vi "Code_generator.vi"(1 "Code":T1(ring)) -> (0 "Array":u16[](array[numeric]) format="%b")   [LabVIEW 2018]
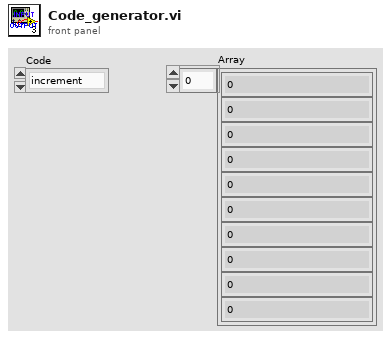
[diagram p1: front panel]
types:
  T1 = enum16{"increment", "decrement", "random", "Chess", "NChess", "One", "Zero"}
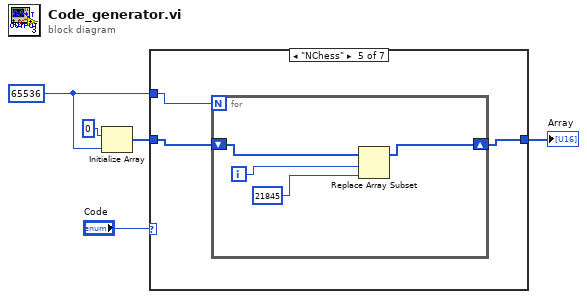
[diagram p0: block diagram]
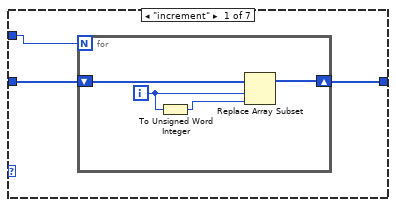
[diagram p2: hidden frame]
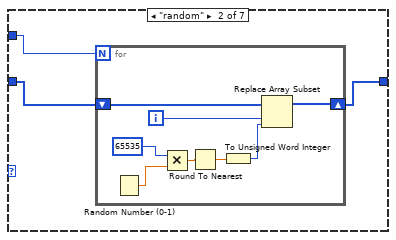
[diagram p3: hidden frame]
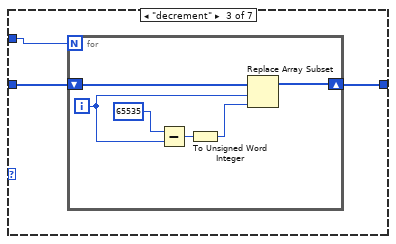
[diagram p4: hidden frame]
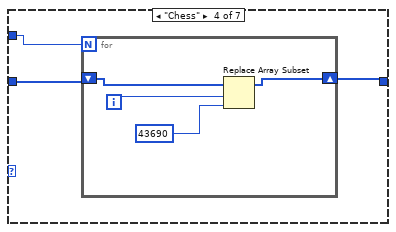
[diagram p5: hidden frame]
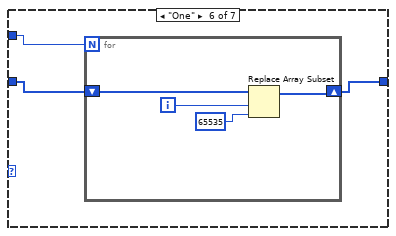
[diagram p6: hidden frame]
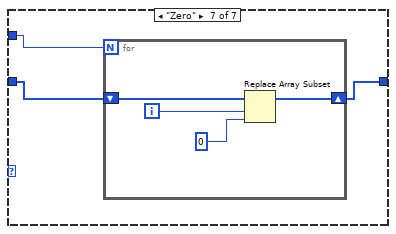
[diagram p7: hidden frame]
diagram:
  w4 = 65536
  n1 = Initialize Array(u16 0, w4) -> (w2:u16[])
  n2 = case shown="\"NChess\"" "Code" {
    tunnel: w4 -> [w8 w15 w26 w35 w42 w49 w56]
    tunnel: w2 -> [w6 w14 w25 w34 w41 w48 w55]
    tunnel: [w7 w13 w24 w33 w40 w47 w54] -> w1
    frame "increment" {
      n3 = for {
        N: w8 -> [_]
        shift-right: [w12] -> w7
        shift-left: w6 -> [w11]
        i -> [w10]
        n4 = To Unsigned Word Integer(number=w10) -> (unsigned 16bit integer=w9:u16)
        n5 = Replace Array Subset(array=w11, new element=w9, index=w10) -> (w12:u16[])
      }
    }
    frame "random" {
      n6 = for {
        N: w15 -> [_]
        shift-right: [w23] -> w13
        shift-left: w14 -> [w22]
        i -> [w21]
        n7 = Random Number (0-1)() -> (number: 0 to 1=w20:dbl)
        n8 = Multiply(x=u16 65535, y=w20) -> (x*y=w18:dbl)
        n9 = Round To Nearest(number=w18) -> (nearest integer value=w16:dbl)
        n10 = To Unsigned Word Integer(number=w16) -> (unsigned 16bit integer=w17:u16)
        n11 = Replace Array Subset(array=w22, new element=w17, index=w21) -> (w23:u16[])
      }
    }
    frame "decrement" {
      n12 = for {
        N: w26 -> [_]
        shift-right: [w32] -> w24
        shift-left: w25 -> [w31]
        i -> [w27]
        n13 = Subtract(x=65535, y=w27) -> (x-y=w29:i32)
        n14 = To Unsigned Word Integer(number=w29) -> (unsigned 16bit integer=w28:u16)
        n15 = Replace Array Subset(array=w31, new element=w28, index=w27) -> (w32:u16[])
      }
    }
    frame "Chess" {
      n16 = for {
        N: w35 -> [_]
        shift-right: [w38] -> w33
        shift-left: w34 -> [w39]
        i -> [w37]
        n17 = Replace Array Subset(array=w39, new element=u16 43690, index=w37) -> (w38:u16[])
      }
    }
    frame "NChess" {
      n18 = for {
        N: w42 -> [_]
        shift-right: [w45] -> w40
        shift-left: w41 -> [w46]
        i -> [w44]
        n19 = Replace Array Subset(array=w46, new element=u16 21845, index=w44) -> (w45:u16[])
      }
    }
    frame "One" {
      n20 = for {
        N: w49 -> [_]
        shift-right: [w53] -> w47
        shift-left: w48 -> [w52]
        i -> [w51]
        n21 = Replace Array Subset(array=w52, new element=u16 65535 ("new element/subarray"), index=w51) -> (w53:u16[])
      }
    }
    frame "Zero" {
      n22 = for {
        N: w56 -> [_]
        shift-right: [w60] -> w54
        shift-left: w55 -> [w59]
        i -> [w58]
        n23 = Replace Array Subset(array=w59, new element=u16 0 ("new element/subarray"), index=w58) -> (w60:u16[])
      }
    }
  }
  "Array" <- w1
